vi "lv_mysql_conn_init_server_data.vi"(8 "error in (no error)":errorcluster, 11 "TCPIP Data":u8[](array[numeric])) -> (0 "error out":errorcluster, 3 "Server Init Data":T1 {"Server Status" format="%.0x"; "Server Languague" format="%.0x"; "Server Capabilities" format="%.0x"})   [LabVIEW 2017]
uses:
  typedefs/server_init_data.ctl
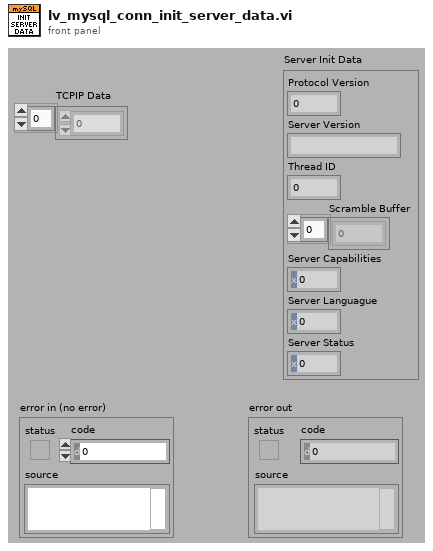
[diagram p1: front panel]
types:
  T1 = typedef "server_init_data.ctl" = cluster{"Protocol Version":u8, "Server Version":string, "Thread ID":u32, "Scramble Buffer":u8[], "Server Capabilities":u16, "Server Languague":u8, "Server Status":u16}
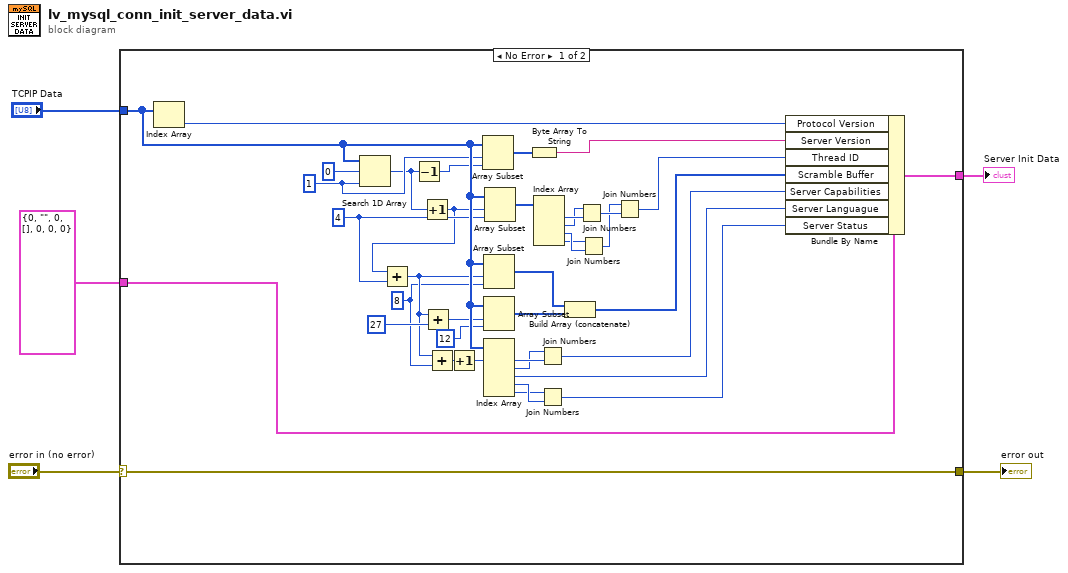
[diagram p0: block diagram]
diagram:
  n1 = case shown="No Error" "error in (no error)" {
    selector: "error in (no error)" -> [w40 w45]
    tunnel: "TCPIP Data" -> [w43 _]
    tunnel: [w42 w44] -> w4
    tunnel: [w40 w45] -> w3
    tunnel: T1 {"Protocol Version"=0, "Server Version"="", "Thread ID"=0, "Scramble Buffer"=[], "Server Capabilities"=0, "Server Languague"=0, "Server Status"=0} ("Server Init Data 2") -> [w39 w44]
    frame No Error {
      w14 = 8 ("length")
      w26 = 4 ("length")
      w37 = 1 ("start index (0)")
      n2 = Index Array(array=w43) -> (element=w41:u8)  [unwired: 1 in]
      n3 = Search 1D Array(1D array=w43, element=u8 0, start index (0)=w37) -> (index of element=w27:i32)
      n4 = Decrement(x=w27) -> (x-1=w35:i32)
      n5 = Increment(x=w27) -> (x+1=w20:i32)
      n6 = Add(x=w20, y=w26) -> (x+y=w15:i32)
      n7 = Add(x=w15, y=27) -> (x+y=w22:i32)
      n8 = Add(x=w15, y=w14) -> (x+y=w13:i32)
      n9 = Increment(x=w13) -> (x+1=w12:i32)
      n10 = Array Subset(array=w43, index=w37, length=w35) -> (w36:u8[])
      n11 = Array Subset(array=w43, index=w15, length=w14) -> (w25:u8[])
      n12 = Array Subset(array=w43, index=w22, length=12) -> (w23:u8[])
      n13 = Index Array(array=w43, index #1=w12) -> (element #1=w19:u8, element #2=w18:u8, element #3=w7:u8, element #4=w17:u8, element #5=w16:u8)  [unwired: 4 in]
      n14 = Array Subset(array=w43, index=w20, length=w26) -> (w34:u8[])
      n15 = Byte Array To String(unsigned byte array=w36) -> (string=w11:string)
      n16 = Index Array(array=w34) -> (element #1=w33:u8, element #2=w32:u8, element #3=w31:u8, element #4=w30:u8)  [unwired: 4 in]
      n17 = Join Numbers(hi=w18, lo=w19) -> ((hi.lo)=w8:u16)
      n18 = Join Numbers(hi=w16, lo=w17) -> ((hi.lo)=w6:u16)
      n19 = Build Array (concatenate)(w25, w23) -> (w9:u8[])
      n20 = Join Numbers(hi=w32, lo=w33) -> ((hi.lo)=w29:u16)
      n21 = Join Numbers(hi=w30, lo=w31) -> ((hi.lo)=w28:u16)
      n22 = Join Numbers(hi=w28, lo=w29) -> ((hi.lo)=w10:u32)
      n23 = Bundle By Name(cluster=w39, "Protocol Version"=w41, "Server Version"=w11, "Thread ID"=w10, "Scramble Buffer"=w9, "Server Capabilities"=w8, "Server Languague"=w7, "Server Status"=w6) -> (w42:T1)
    }
    frame Error {
    }
  }
  "Server Init Data" <- w4
  "error out" <- w3
